vi "Rotate 2D velocity vector.vi"(3 "V":dbl, 4 "U":dbl, 5 "Rotation angle (deg)":dbl) -> (0 "V~":dbl, 1 "U~":dbl)   [LabVIEW 2014]
panel:
  # "Anti-clockwise looking into axis of rotation. Rotation is about the axis perpendicular to the plane of the measured velocity vector."
  # "Components must be coincident samples!"
  # "PN 21/10/2014"
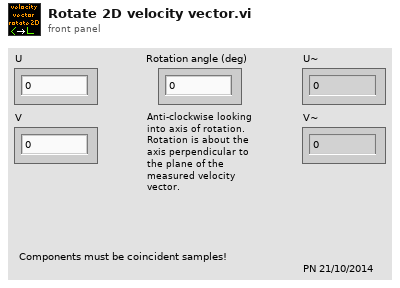
[diagram p1: front panel]
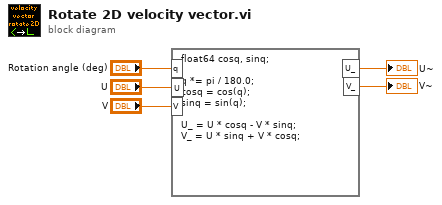
[diagram p0: block diagram]
diagram:
  n1 = formula code="float64 cosq, sinq;\n\nq *= pi / 180.0;\ncosq = cos(q);\nsinq = sin(q);\n\nU_ = U * cosq - V * sinq;\nV_ = U * sinq + V * cosq;"("U"="U", "V"="V", "q"="Rotation angle (deg)") -> ("U_"=→"U~":dbl, "V_"=→"V~":dbl)
